vi "List columns.vi"(8 "error in (no error)":errorcluster, 10 "table":string, 11 "database":string="database1.mdb") -> (0 "error out":errorcluster, 3 "columns":string[](array[string]))   [LabVIEW 2016, in "数据查询.lvlib"]
uses:
  <vilib>/addons/database/Connection.llb/DB Tools Open Connec (String).vi
  <userlib>/_LVST/sqlite_api/Core/Tables/SQLite_List Columns.vi
  <vilib>/addons/database/NI_Database_API.lvlib
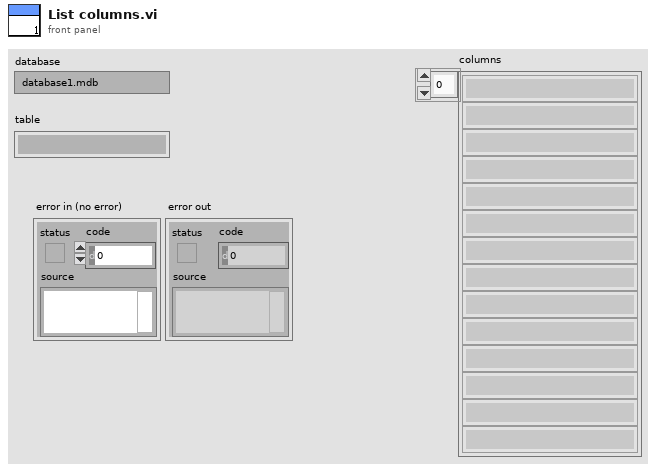
[diagram p1: front panel]
types:
  T1 = typedef "NI_Database_API.lvlib/Conn ObjectReference.ctl" = refnum<k1>
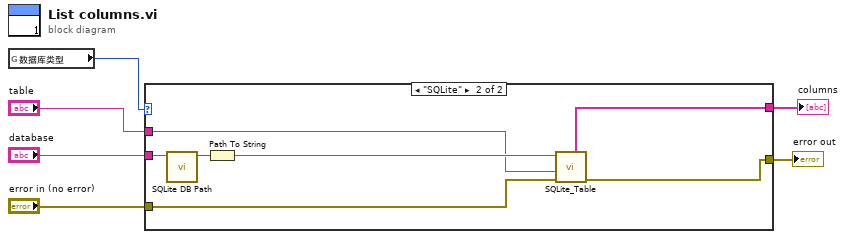
[diagram p0: block diagram]
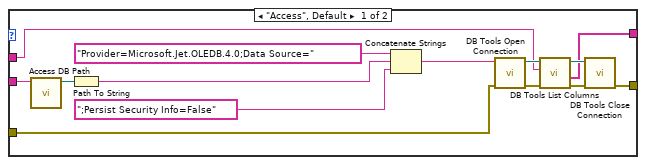
[diagram p2: hidden frame]
diagram:
  n1 = global read "全局变量.vi" "数据库类型"() -> (w1:enum16{"Access", "SQLite"})
  n2 = case shown="\"SQLite\"" w1 {
    tunnel: "table" -> [w16 w24]
    tunnel: "error in (no error)" -> [w15 w21]
    tunnel: [w14 w22] -> w4
    tunnel: "database" -> [w9 w27]
    tunnel: [w7 w23] -> w2
    frame "Access", Default {
      n3 = call "Access DB Path.vi"("database"=w9) -> ("appended path"=w8:path)  [unwired: 10 in]
      n4 = Path To String(path=w8) -> (string=w12:string)
      n5 = Concatenate Strings("Provider=Microsoft.Jet.OLEDB.4.0;Data Source=" ("condition"), w12, ";Persist Security Info=False" ("condition")) -> (w10:string)
      n6 = call-poly <vilib>:"DB Tools Open Connection.vi"("error in (no error)"=w15, "connection information"=w10) -> ("error out"=w18:errorcluster, "connection reference"=w20:T1)  [unwired: 6 in]
      n7 = call <vilib>:"DB Tools List Columns.vi"("error in (no error)"=w18, "table"=w16, "connection reference"=w20) -> ("error out"=w17:errorcluster, "columns"=w7:string[], "connection reference out"=w19:T1)  [unwired: 1 in, 1 out]
      n8 = call <vilib>:"DB Tools Close Connection.vi"("error in (no error)"=w17, "connection reference"=w19) -> ("error out"=w14:errorcluster)  [unwired: 5 in]
    }
    frame "SQLite" {
      n9 = call "SQLite DB Path.vi"("database"=w27) -> ("appended path"=w25:path)  [unwired: 10 in]
      n10 = Path To String(path=w25) -> (string=w26:string)
      n11 = call-poly <userlib>:"SQLite_Table.vi"("DB Path"=w26, "Table Name"=w24, "error in (no error)"=w21) -> ("Columns"=w23:string[], "error out"=w22:errorcluster)  [unwired: 4 in, 2 out]
    }
  }
  "error out" <- w4
  "columns" <- w2
